vi "Filter RX signals.vi"(0 "Symbols":cdb[](array[numeric]) format="%.2f", 1 "Samples Per Symbol (16)":i32=16, 2 "RX Matched Filter Coefficients":dbl[](array[numeric]) format="%.2f", 3 "Number of Symbols":i32, 4 "TX Pulse Shaping Filter Coefficients":dbl[](array[numeric]) format="%.2f") -> (7 "decimated symbols":cdb[](array[numeric]) caption="Filtered Samples" format="%.2f", 10 "Filtered Samples":cdb[](array[numeric]))   [LabVIEW 2011]
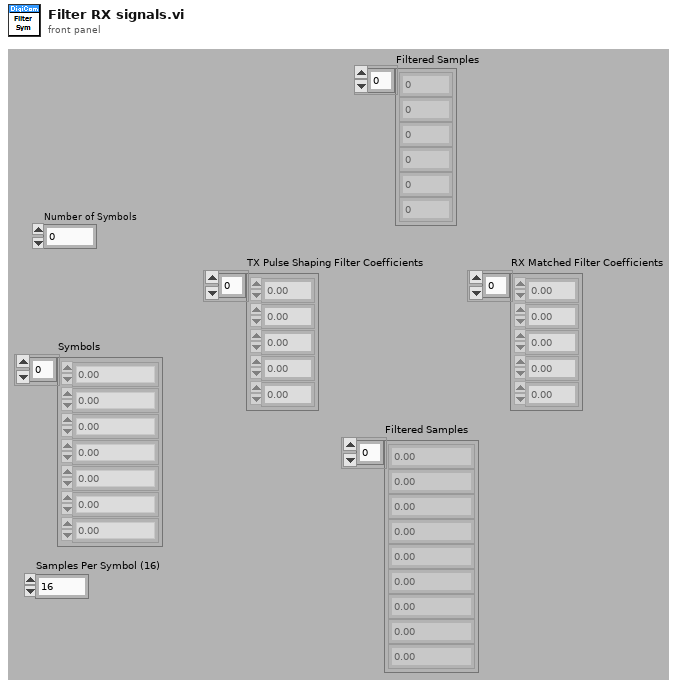
[diagram p1: front panel]
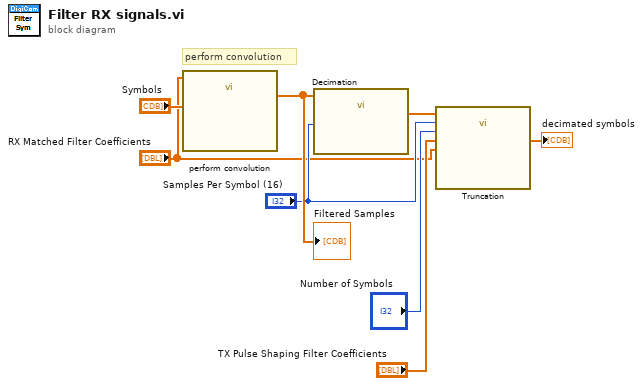
[diagram p0: block diagram]
diagram:
  # "perform convolution"
  n1 = call "perform convolution.vi"("Sample stream"="Symbols", "Pulse Shaping Filter Coefficients"="RX Matched Filter Coefficients") -> ("Filtered sample stream"=w7:cdb[])  [unwired: 9 in]
  "Filtered Samples" <- w7
  n2 = call "Decimation.vi"("Samples per Symbol"="Samples Per Symbol (16)", "Signal In"=w7) -> ("Signal Out"=w5:cdb[])  [unwired: 9 in]
  n3 = call "Truncation.vi"("original signals"=w5, "Samples Per Symbol (16)"="Samples Per Symbol (16)", "Number of Symbols"="Number of Symbols", "TX Pulse Shaping Filter Coefficients"="TX Pulse Shaping Filter Coefficients", "RX Matched Filter Coefficients"="RX Matched Filter Coefficients") -> ("truncated signals"=→"decimated symbols":cdb[])  [unwired: 10 in]
